vi "Average Trailing.vi"(2 "averg #":dbl=0.95, 3 "Input":dbl, 4 "Previous\nValue":dbl) -> (1 "Output":dbl)   [LabVIEW 2013]
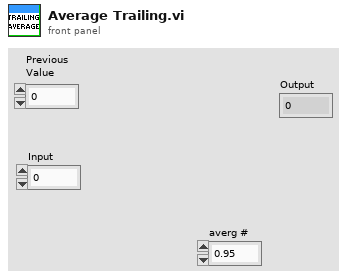
[diagram p1: front panel]
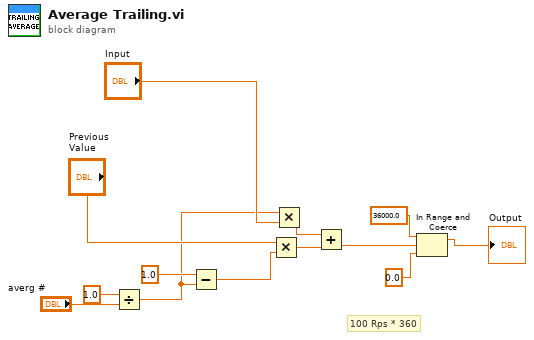
[diagram p0: block diagram]
diagram:
  # "100 Rps * 360"
  n1 = Divide(x=1.0, y="averg #") -> (x/y=w6:dbl)
  n2 = Subtract(x=1.0, y=w6) -> (x-y=w5:dbl)
  n3 = Multiply(x="Previous\nValue", y=w5) -> (x*y=w13:dbl)
  n4 = Multiply(x=w6, y="Input") -> (x*y=w12:dbl)
  n5 = Add(x=w12, y=w13) -> (x+y=w4:dbl)
  n6 = In Range and Coerce(upper limit=36000.0, x=w4, lower limit=0.0) -> (coerced(x)=→"Output":dbl)  [unwired: 1 out]
